vi "mono-Isport.vi"(8 "error in (no error)":errorcluster, 11 "Monochromator":refnum<vi>) -> (0 "Error Out":errorcluster, 2 "Boolean":bool, 3 "Monochromator out":refnum<vi>)   [LabVIEW 2016]
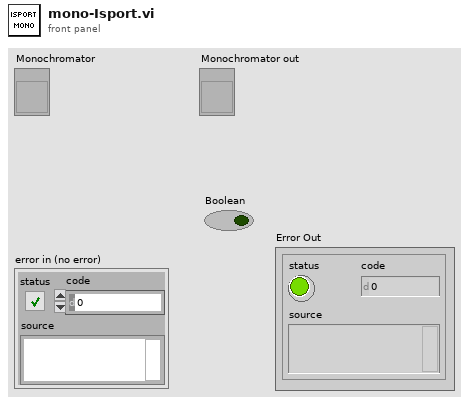
[diagram p1: front panel]
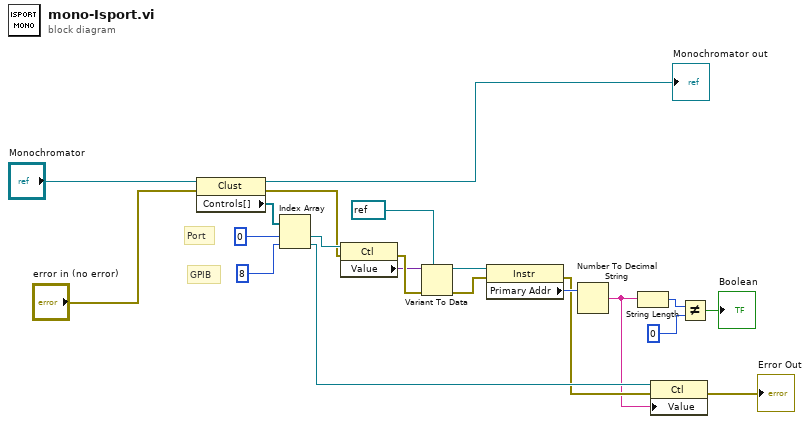
[diagram p0: block diagram]
diagram:
  # "GPIB"
  # "Port"
  n1 = property class="Clust"(reference="Monochromator", error in="error in (no error)") -> (reference out=→"Monochromator out":refnum<vi>, error out=w12:errorcluster, "Controls[]"=w15:refnum<vi>[])
  n2 = Index Array(array=w15, index #1=0 ("index"), index #2=8 ("index")) -> (element #1=w13:refnum<vi>, element #2=w4:refnum<vi>)
  n3 = property class="Ctl"(reference=w13, error in=w12) -> (error out=w11:errorcluster, "Value"=w10:variant)  [unwired: 1 out]
  n4 = Variant To Data(error in=w11, type=refnum<visa-resource-name> refnum ("reference out"), Variant=w10) -> (data=w8:refnum<visa-resource-name>, error out=w6:errorcluster)
  n5 = property class="Instr"(reference=w8, error in=w6) -> (error out=w3:errorcluster, "Primary Addr"=w7:u16)  [unwired: 1 out]
  n6 = Number To Decimal String(number=w7) -> (decimal integer string=w2:string)  [unwired: 1 in]
  n7 = String Length(string=w2) -> (length=w16:i32)
  n8 = property class="Ctl"(reference=w4, error in=w3, "Value"=w2) -> (error out=→"Error Out":errorcluster)  [unwired: 1 out]
  n9 = Not Equal?(x=w16, y=0) -> (x != y?=→"Boolean":bool)
